vi "worksheet merge range lv.vi"(4 "format":u32, 5 "string":string, 6 "last_col":u16, 7 "last_row":u32, 8 "error in (no error)":errorcluster, 9 "first_col":u16, 10 "first_row":u32, 11 "worksheet":u32) -> (0 "error out":errorcluster, 3 "function return":u32(ring))   [LabVIEW 8.6]
doc: "lxw_error worksheet_merge_range_lv(lxw_worksheet worksheet, lxw_row_t first_row, lxw_col_t first_col, lxw_row_t last_row, lxw_col_t last_col, const char *string, lxw_format format);"
uses:
  pending_lvxlsxwriter/xlsxwriter.dll
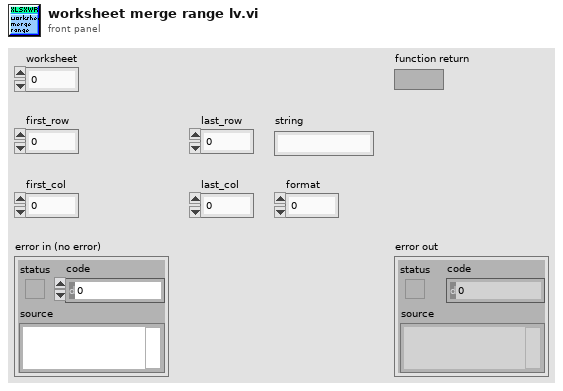
[diagram p1: front panel]
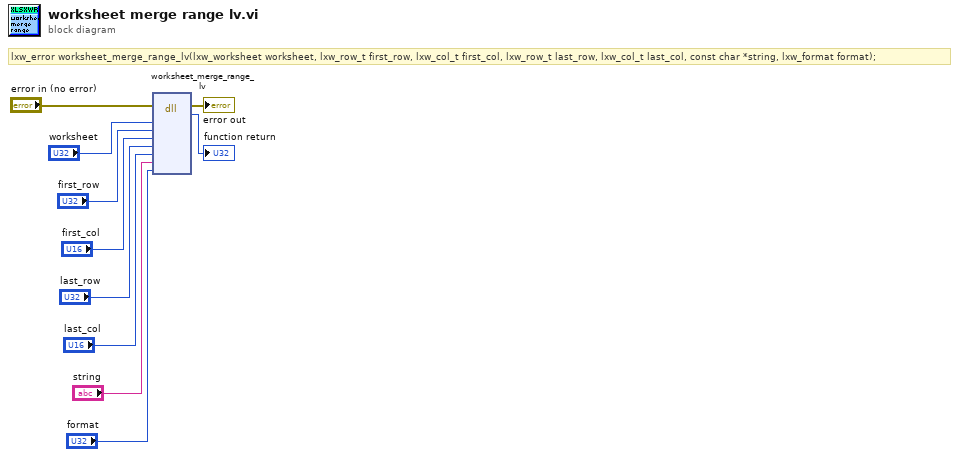
[diagram p0: block diagram]
diagram:
  # "lxw_error worksheet_merge_range_lv(lxw_worksheet worksheet, lxw_row_t first_row, lxw_col_t first_col, lxw_row_t last_row, lxw_col_t last_col, const char *string, lxw_format format);"
  n1 = dll-call lib="C:/Users/WDAGUtilityAccount/Desktop/pending_lvxlsxwriter/xlsxwriter.*" fn="worksheet_merge_range_lv"(error in="error in (no error)", "worksheet"="worksheet", "first_row"="first_row", "first_col"="first_col", "last_row"="last_row", "last_col"="last_col", "string"="string", "format"="format") -> (error out=→"error out":errorcluster, →"function return":u32)  [unwired: 9 in, 1 out]
